vi "Pressure pulse.vi"(8 "error in (no error)":errorcluster, 10 "Up or down?":enum16{"Up", "Down"}(ring), 11 "Pressure Control in":refnum<class "Pressure Control.lvclass">) -> (0 "error out":errorcluster, 3 "Pressure Control out":refnum<class "Pressure Control.lvclass">)   [LabVIEW 2011, in "Pressure Control.lvclass"]
doc: "Gives a TTL pulse, either to the \"Pressure up\" or the \"Pressure down\" line"
uses:
  Pressure Control.lvclass
  Pressure Control.lvclass/Pressure Control.ctl
  TTL/TTL.lvclass
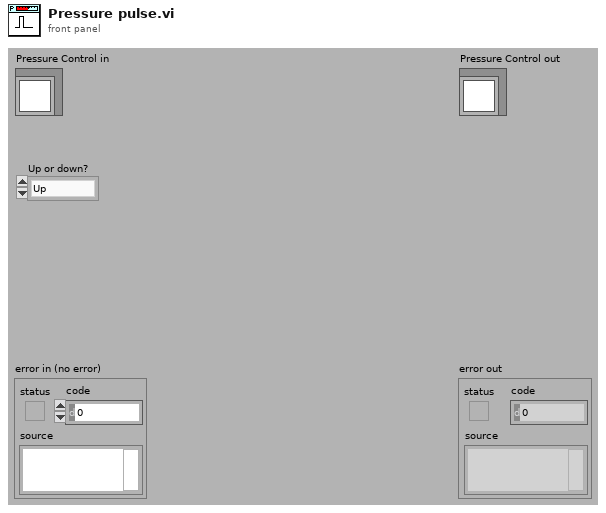
[diagram p1: front panel]
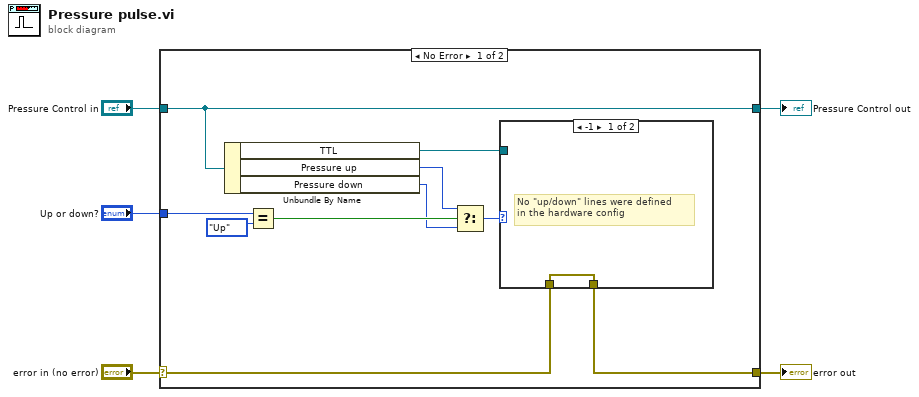
[diagram p0: block diagram]
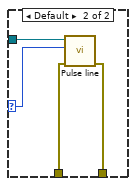
[diagram p2: hidden frame]
diagram:
  n1 = case shown="No Error" "error in (no error)" {
    selector: "error in (no error)" -> [w8 w22]
    tunnel: [w7 w22] -> w4
    tunnel: [w15 w21] -> w2
    tunnel: "Pressure Control in" -> [w15 w21]
    tunnel: "Up or down?" -> [w14 _]
    frame No Error {
      n2 = Unbundle By Name(w15) -> ("TTL"=w9:refnum<class "TTL.lvclass">, "Pressure up"=w11:i32, "Pressure down"=w10:i32)
      n3 = Equal?(x=w14, y=enum16{"Up", "Down"}."Up") -> (x = y?=w12:bool)
      n4 = Select(t=w11, s=w12, f=w10) -> (s? t:f=w6:i32)
      n5 = case shown="-1" w6 {
        selector: w6 -> [_ w17]
        tunnel: w9 -> [_ w20]
        tunnel: w8 -> [w16 w19]
        tunnel: [w16 w18] -> w7
        frame -1 {
          # "No \"up/down\" lines were defined\nin the hardware config"
        }
        frame Default {
          n6 = call "Pulse line.vi"("error in (no error)"=w19, "Line number"=w17, "TTL in"=w20) -> ("error out"=w18:errorcluster)  [unwired: 7 in, 1 out]
        }
      }
    }
    frame Error {
    }
  }
  "error out" <- w4
  "Pressure Control out" <- w2
